vi "Set Force Sensor Settings.vi"(10 "Force Sensor Settings":T1={"Reference Voltage Vref"=0.0, "Force Sensor Calculator"={"Capacity"=1.0, "Sensitivity"=0.001}} {"Force Sensor Calculator"."Sensitivity" min=0.001 max=5000.0 format="%.4f"; "Force Sensor Calculator"."Capacity" min=1.0 max=5000000.0 format="%.4f"; "Reference Voltage Vref" min=-10.0 max=10.0 format="%.3f"}, 11 "Tovey9150 in":refnum<class "Tovey 9150.lvclass">) -> (3 "Tovey9150 out":refnum<class "Tovey 9150.lvclass">)   [LabVIEW 2015]
uses:
  Tovey 9150.lvclass
  <userlib>/Common/Devices/ForceSensorCalculator/Config/ForceSensorCalculator.ctl
  <userlib>/Common/Devices/ForceSensorCalculator/ForceSensorCalculator.lvlib
  Typedefs/Force Sensor Settings.ctl
  Typedefs/FAMT Typedefs.lvlib
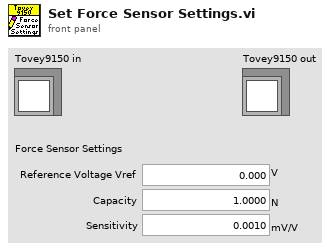
[diagram p1: front panel]
types:
  T1 = typedef "FAMT Typedefs.lvlib/Force Sensor Settings.ctl" = cluster{"Reference Voltage Vref":dbl[unit], "Force Sensor Calculator":T2}
  T2 = typedef "ForceSensorCalculator.lvlib/ForceSensorCalculator.ctl" = cluster{"Capacity":dbl[unit], "Sensitivity":dbl[unit]}
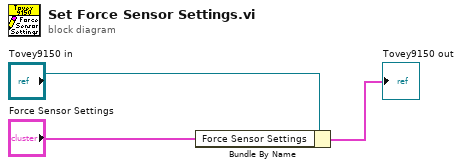
[diagram p0: block diagram]
diagram:
  n1 = Bundle By Name(cluster="Tovey9150 in", "Force Sensor Settings"="Force Sensor Settings") -> (→"Tovey9150 out":cluster{})
